vi "Calc imei checkdigit.vi"(8 "error in (no error)":errorcluster, 11 "14 digit IMEI":string) -> (0 "error out":errorcluster, 2 "15 digit imei":string, 3 "15 digit imei ok?":bool)   [LabVIEW 2013]
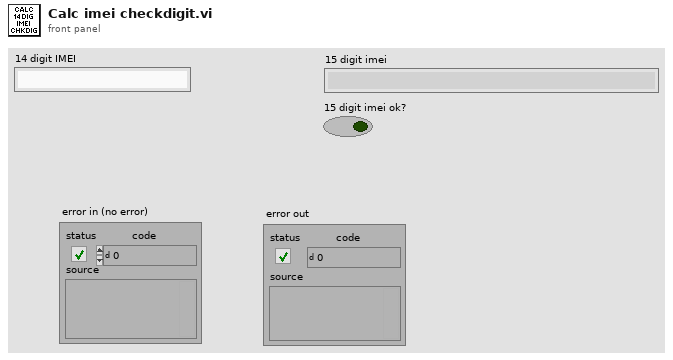
[diagram p1: front panel]
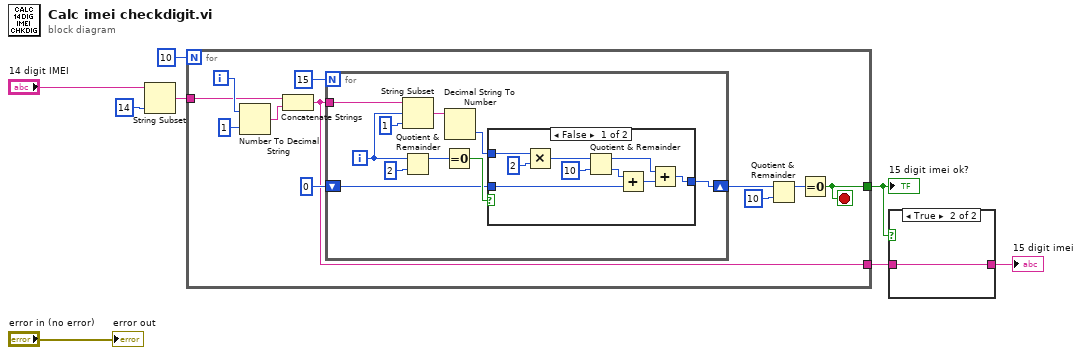
[diagram p0: block diagram]
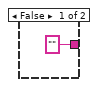
[diagram p2: hidden frame]
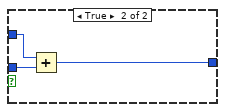
[diagram p3: hidden frame]
diagram:
  n1 = String Subset(string="14 digit IMEI", length (rest)=14 ("length (rest)")) -> (substring=w5:string)  [unwired: 1 in]
  n2 = for {
    N: 10 -> [_]
    tunnel: w5 -> [w13]
    tunnel: [w11] -> w7
    tunnel: [w10] -> w6
    i -> [w14]
    stop <- w11 stop-if-true
    n3 = Number To Decimal String(number=w14, width (-)=i16 1) -> (decimal integer string=w12:string)
    n4 = Concatenate Strings(w13, w12) -> (w10:string)
    n5 = for {
      N: 15 -> [_]
      tunnel: w10 -> [w29]
      shift-right: [w20] -> w17
      shift-left: 0 -> [w21]
      i -> [w27]
      n6 = String Subset(string=w29, offset (0)=w27, length (rest)=1 ("length (rest)")) -> (substring=w23:string)
      n7 = Quotient & Remainder(x=w27, y=2) -> (x-y*floor(x/y)=w25:i32)  [unwired: 1 out]
      n8 = Equal To 0?(x=w25) -> (x = 0?=w24:bool)
      n9 = Decimal String To Number(string=w23) -> (number=w22:i32)  [unwired: 2 in, 1 out]
      n10 = case shown="False" w24 {
        tunnel: w22 -> [w38 w41]
        tunnel: w21 -> [w33 w40]
        tunnel: [w30 w39] -> w20
        frame False {
          n11 = Multiply(x=w38, y=2) -> (x*y=w36:i32)
          n12 = Quotient & Remainder(x=w36, y=10) -> (x-y*floor(x/y)=w32:i32, floor(x/y)=w34:i32)
          n13 = Add(x=w34, y=w33) -> (x+y=w31:i32)
          n14 = Add(x=w32, y=w31) -> (x+y=w30:i32)
        }
        frame True {
          n15 = Add(x=w41, y=w40) -> (x+y=w39:i32)
        }
      }
    }
    n16 = Quotient & Remainder(x=w17, y=10) -> (x-y*floor(x/y)=w15:i32)  [unwired: 1 out]
    n17 = Equal To 0?(x=w15) -> (x = 0?=w11:bool)
  }
  "15 digit imei ok?" <- w7
  n18 = case shown="True" w7 {
    tunnel: w6 -> [_ w43]
    tunnel: ["" w43] -> w8
    frame False {
    }
    frame True {
    }
  }
  "15 digit imei" <- w8
  "error out" <- "error in (no error)"
